vi "dotNET Parse Measurement Details.vi"(8 "error in":errorcluster) -> (0 "error out":errorcluster, 3 "Measurement Meta Details":T1)   [LabVIEW 2020, in "Measurement Client Wrapper.lvclass"]
uses:
  Measurement Client Wrapper.lvclass
  Typedefs/Measurement meta details.ctl
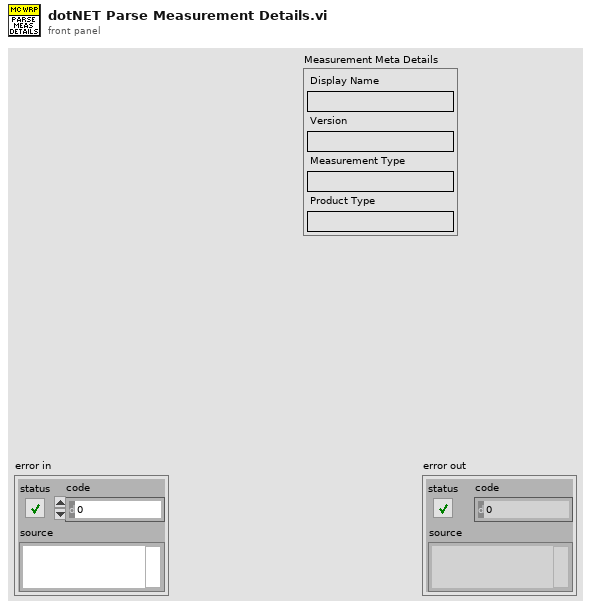
[diagram p1: front panel]
types:
  T1 = typedef "Measurement meta details.ctl" = cluster{"Display Name":string, "Version":string, "Measurement Type":string, "Product Type":string}
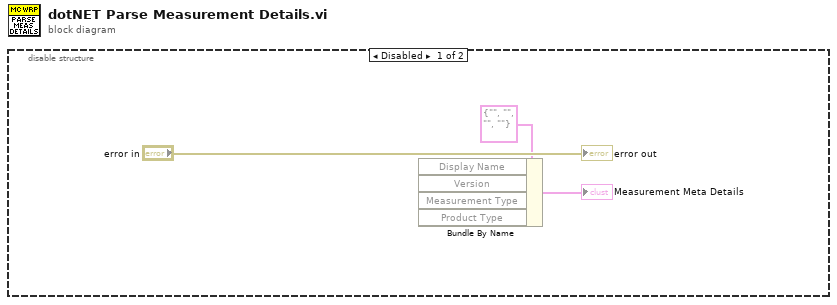
[diagram p0: block diagram]
diagram:
  n1 = disable-structure shown="Disabled" {
    frame Disabled {
      n2 = Bundle By Name(cluster=T1 {"Display Name"="", "Version"="", "Measurement Type"="", "Product Type"=""} ("Measurement Meta Details")) -> (→"Measurement Meta Details":T1)  [unwired: 4 in]
      "error out" <- "error in"
    }
    frame Enabled {
    }
  }
